vi "setDevices.vi"(8 "error in (no error)":errorcluster, 10 "Devices":refnum<class "ACNET Device.lvclass">[](array[class]), 11 "ACNET Devices in":refnum<class "ACNET Devices.lvclass">) -> (0 "error out":errorcluster, 3 "ACNET Devices out":refnum<class "ACNET Devices.lvclass">)   [LabVIEW 2013, in "ACNET Monitor.lvlib" / "ACNET Devices.lvclass"]
uses:
  ACNET Devices.lvclass
  ACNET Device.lvclass
  ACNET Devices.lvclass/ACNET Devices.ctl
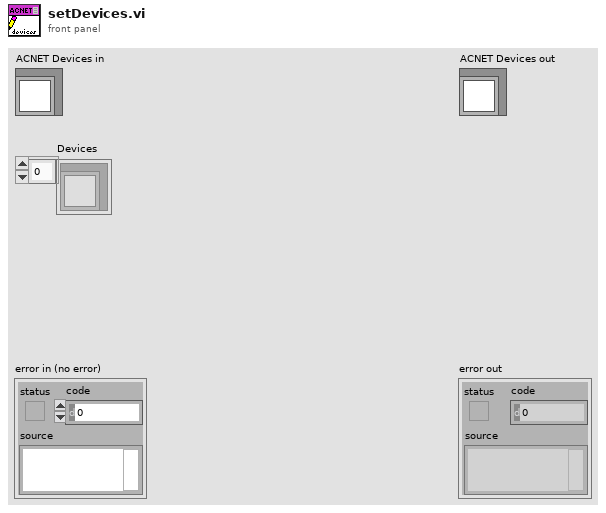
[diagram p1: front panel]
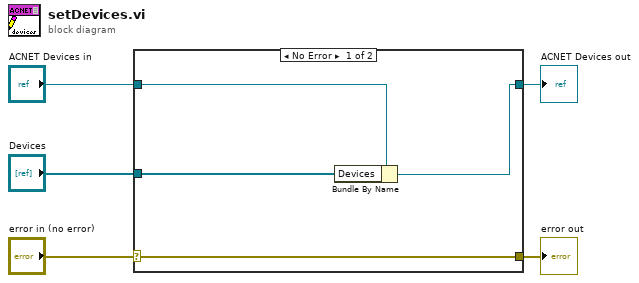
[diagram p0: block diagram]
diagram:
  n1 = case shown="No Error" "error in (no error)" {
    selector: "error in (no error)" -> [w9 w10]
    tunnel: [w9 w10] -> w4
    tunnel: [w7 w11] -> w2
    tunnel: "ACNET Devices in" -> [w8 w11]
    tunnel: "Devices" -> [w6 _]
    frame No Error {
      n2 = Bundle By Name(cluster=w8, "Devices"=w6) -> (w7:refnum<class "ACNET Devices.lvclass">)
    }
    frame Error {
    }
  }
  "error out" <- w4
  "ACNET Devices out" <- w2
